vi "File Transfare.vi"(8 "Error In":errorcluster, 9 "Target File Path":string="ni-rt/Bowl.gcode", 10 "Local File Path":path=path "C:/3D Printer Project/Support Files/Bowl.gcode", 11 "Host Addess":string="http://10.92.1.42/files/") -> (0 "Error Out":errorcluster)   [LabVIEW 2018]
uses:
  <vilib>/WebDAVClient/Advanced/Put File.vi
  <vilib>/WebDAVClient/NI_WebDAV.lvlib
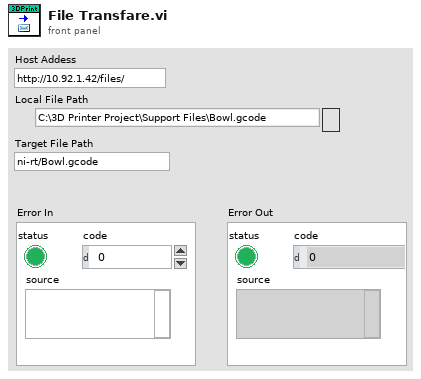
[diagram p1: front panel]
types:
  T1 = typedef "NI_WebDAV.lvlib/SessionHandle.ctl" = refnum<k1>
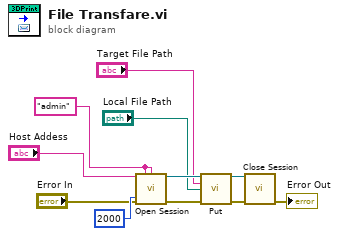
[diagram p0: block diagram]
diagram:
  w11 = "admin" ("username")
  n1 = call <vilib>:"Open Session.vi"("host uri prefix"="Host Addess", "username"=w11, "password"=w11, "error in (no error)"="Error In", "timeout ms"=2000) -> ("session handle out"=w7:T1, "error out"=w8:errorcluster)  [unwired: 9 in]
  n2 = call-poly <vilib>:"Put.vi"("session handle"=w7, "relative uri"="Target File Path", "local file path"="Local File Path", "error in (no error)"=w8) -> ("session handle out"=w2:T1, "error out"=w1:errorcluster)  [unwired: 9 in, 1 out]
  n3 = call <vilib>:"Close Session.vi"("session handle"=w2, "error in (no error)"=w1) -> ("error out"=→"Error Out":errorcluster)  [unwired: 13 in]
